vi "trivial_req.vi"(8 "error in":errorcluster, 10 "data to send":string="hello", 11 "endpoint":string="tcp://127.0.0.1:5555") -> (0 "error out":errorcluster, 2 "reply":string)   [LabVIEW 2018]
uses:
  LV-Julia_ZMQ-Roundtrip_lib.lvlib
panel:
  out "more?":bool
  out "timeout?":bool
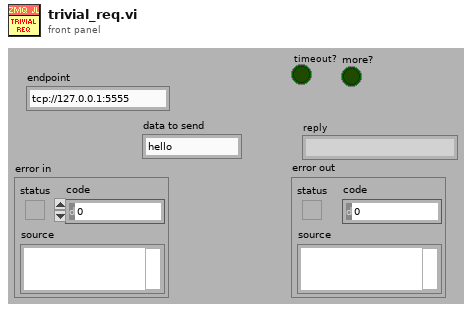
[diagram p1: front panel]
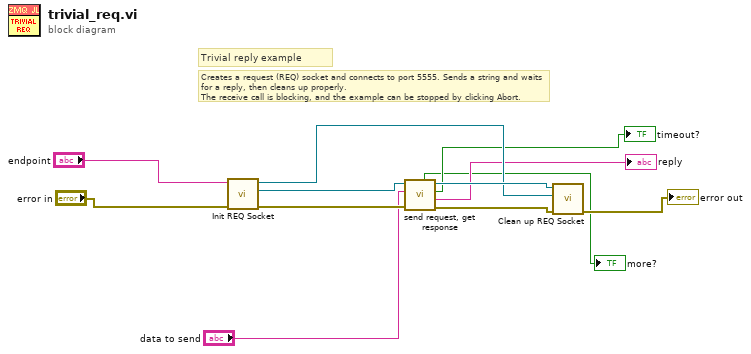
[diagram p0: block diagram]
diagram:
  # "Creates a request (REQ) socket and connects to port 5555. Sends a string and waits for a reply, then cleans up properly.\nThe receive call is blocking, and the example can be stopped by clicking Abort."
  # "Trivial reply example"
  n1 = call "Init REQ Socket.vi"("error in (no error)"="error in", "endpoint"="endpoint") -> ("error out"=w12:errorcluster, "socket out"=w11:refnum<class "zmq_socket.lvclass">, "zmq_context out"=w8:refnum<class "zmq_context.lvclass">)  [unwired: 7 in]
  n2 = call "send request, get response.vi"("error in (no error)"=w12, "request"="data to send", "zmq_socket in"=w11) -> ("error out"=w10:errorcluster, "response"=→"reply":string, "timeout?"=→"timeout?":bool, "zmq_socket out"=w9:refnum<class "zmq_socket.lvclass">, "more?"=→"more?":bool)  [unwired: 4 in]
  n3 = call "Clean up REQ Socket.vi"("error in (no error)"=w10, "zmq_context in"=w8, "zmq_socket in"=w9) -> ("error out"=→"error out":errorcluster)  [unwired: 8 in]
